vi "Wait_Darker_Step1.vi"   [LabVIEW 2012]
uses:
  <vilib>/NXT/Subs/MotorOutput.ctl
  <vilib>/NXT/Block Support/NXT_InputPort.ctl
types:
  T1 = typedef "NXT_InputPort.ctl" = u32
  T2 = typedef "MotorOutput.ctl" = u8
  T3 = typedef "LVHSConnector.ctl" = refnum<class "BrickReference.lvclass">
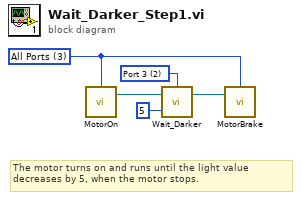
[diagram p0: block diagram]
diagram:
  w1 = T1 2 items=["Port 1", "Port 2", "Port 3", "Port 4"] ("Port (Port 3)")
  w3 = T2 3 items=["Port A", "Port B", "Port C", "All Ports"] ("Output Port")
  # "The motor turns on and runs until the light value\ndecreases by 5, when the motor stops."
  n1 = call <vilib>:"MotorOn.vi"("Output Port (All Ports)"=w3) -> ("NXT/EV3"=w5:T3)  [unwired: 3 in]
  n2 = call <vilib>:"Wait_Darker.vi"("Darker (5)"=u8 5 ("Brightness Change (5)"), "NXT/EV3"=w5, "Port (Port 3)"=w1) -> ("NXT/EV3"=w4:T3)  [unwired: 1 in]
  n3 = call <vilib>:"MotorBrake.vi"("NXT/EV3"=w4, "Port (All Ports)"=w3) -> ()  [unwired: 2 in, 1 out]
